vi "BlendSuggestionsToTurn.vi"(10 "SailsByTurningBoat":T1 {"MainSailSuggestion" min=0.0 max=1.0; "JibSailSuggestion" min=0.0 max=1.0}, 11 "WindToSailLookup":T1 {"MainSailSuggestion" min=0.0 max=1.0; "JibSailSuggestion" min=0.0 max=1.0}) -> (3 "BlendedTurningSailSetting":T1 {"MainSailSuggestion" min=0.0 max=1.0; "JibSailSuggestion" min=0.0 max=1.0})   [LabVIEW 2013]
doc: "This VI takes in suggestions for\n1) Simple sail lookup by Point of Sail\n2) How to move the sails to balance the rudder\n3) How to move the sails to stop luffing\n\nThis VI is intended to generally pass through #1 unimpeded, but gradually filter in the advice from #2 and #3 over time. The mechanism for this will be either increasing the gain of suggestions (2, 3) as the boat nears 'cruising' velocity or indcreasing the gain as a function of the time spent in the 'go straight' boat state."
uses:
  Data/TypeDefs/Sail Set Suggestions.ctl
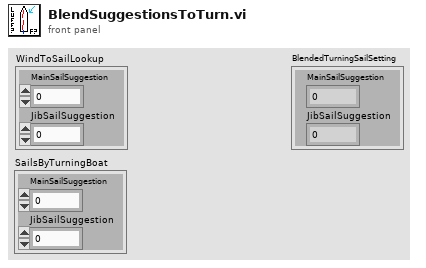
[diagram p1: front panel]
types:
  T1 = typedef "Sail Set Suggestions.ctl" = cluster{"MainSailSuggestion":dbl, "JibSailSuggestion":dbl}
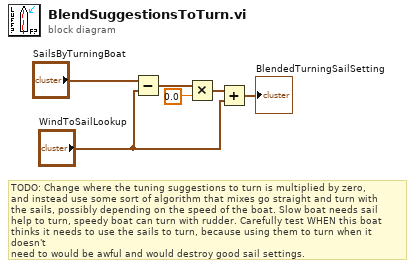
[diagram p0: block diagram]
diagram:
  # "TODO: Change where the tuning suggestions to turn is multiplied by zero,\nand instead use some sort of algorithm that mixes go straight and turn with\nthe sails, possibly depending on the speed of the boat. Slow boat needs sail\nhelp to turn, speedy boat can turn with rudder. Carefully test WHEN this boat\nthinks it needs to use the sails to turn, because using them to turn when it doesn't\nneed to would be awful and would destroy good sail settings."
  n1 = Subtract(x="SailsByTurningBoat", y="WindToSailLookup") -> (x-y=w6:T1)
  n2 = Multiply(x=w6, y=0.0) -> (x*y=w2:T1)
  n3 = Add(x=w2, y="WindToSailLookup") -> (x+y=→"BlendedTurningSailSetting":T1)
